vi "Read Data Rigol.vi"(7 "error in (no error)":errorcluster, 9 "CH number":i32, 10 "VISA resource name":refnum<visa-resource-name>) -> (0 "error out":errorcluster, 1 "Actual Current Level (A)":dbl caption="Actual Current Level" format="%.2f", 2 "Actual Voltage Level (V)":dbl caption="Actual Voltage Level" format="%.2f", 3 "VISA resource name out":refnum<visa-resource-name>)   [LabVIEW 2023, in "Rigol.lvlib"]
uses:
  <instrlib>/RIGOL DP800 Series/Public/Channels.ctl
  Rigol.lvlib
  <instrlib>/RIGOL DP800 Series/RIGOL DP800 Series.lvlib
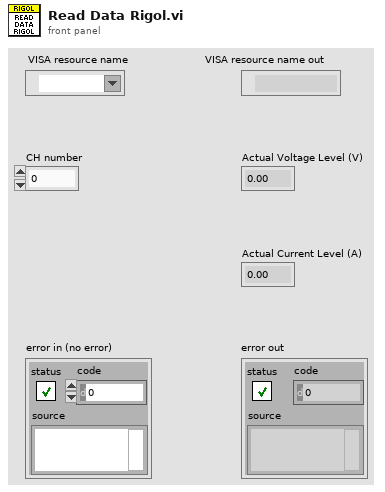
[diagram p1: front panel]
types:
  T1 = typedef "RIGOL DP800 Series.lvlib/Channels.ctl" = i32
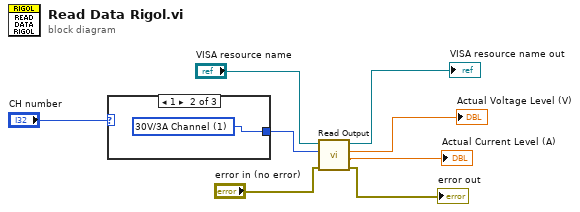
[diagram p0: block diagram]
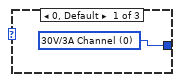
[diagram p2: hidden frame]
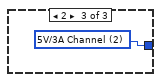
[diagram p3: hidden frame]
diagram:
  n1 = case shown="1" "CH number" {
    tunnel: [w9 w10 w11] -> w3
    frame 0, Default {
      w9 = T1 0 items=["30V/3A Channel", "30V/3A Channel", "5V/3A Channel"] ("Channel (0: 30V Channel)")
    }
    frame 1 {
      w10 = T1 1 items=["30V/3A Channel", "30V/3A Channel", "5V/3A Channel"] ("Channel (0: 30V Channel)")
    }
    frame 2 {
      w11 = T1 2 items=["30V/3A Channel", "30V/3A Channel", "5V/3A Channel"] ("Channel (0: 30V Channel)")
    }
  }
  n2 = call <instrlib>:"Read Output.vi"("error in (no error)"="error in (no error)", "Channel (0: 30V Channel)"=w3, "VISA resource name"="VISA resource name") -> ("error out"=→"error out":errorcluster, "Actual Current Level (A)"=→"Actual Current Level (A)":dbl, "Actual Voltage Level (V)"=→"Actual Voltage Level (V)":dbl, "VISA resource name out"=→"VISA resource name out":refnum<visa-resource-name>)  [unwired: 4 in, 1 out]
